vi "Set FP Origin.vi"(8 "error in":errorcluster, 11 "VI ref in":refnum<vi>) -> (0 "error out":errorcluster, 3 "VI Ref out":refnum<vi>)   [LabVIEW 2021, in "Utility.lvlib"]
uses:
  Utility.lvlib
  <vilib>/Utility/miscctls.llb/LVPointTypeDef.ctl
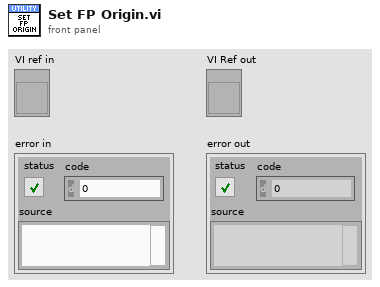
[diagram p1: front panel]
types:
  T1 = typedef "LVPointTypeDef.ctl" = cluster{"Horizontal":i16, "Vertical":i16}
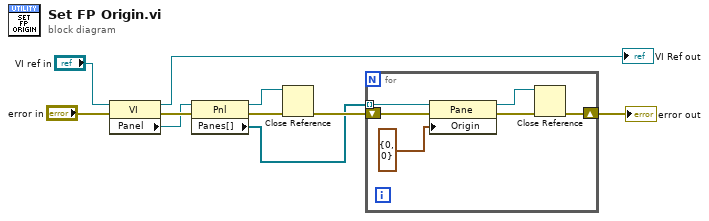
[diagram p0: block diagram]
diagram:
  n1 = property class="VI"(reference="VI ref in", error in="error in") -> (reference out=→"VI Ref out":refnum<vi>, error out=w6:errorcluster, "Panel"=w3:refnum<vi>)
  n2 = property class="Pnl"(reference=w3, error in=w6) -> (reference out=w4:refnum<vi>, error out=w8:errorcluster, "Panes[]"=w2:refnum<vi>[])
  n3 = Close Reference(reference=w4, error in (no error)=w8) -> (error out=w9:errorcluster)
  n4 = for {
    tunnel: w2 -> [w13] mode=indexing
    shift-right: [w14] -> w10
    shift-left: w9 -> [w16]
    n5 = property class="Pane"(reference=w13, error in=w16, "Origin"=T1 {"Horizontal"=0, "Vertical"=0}) -> (reference out=w11:refnum<vi>, error out=w15:errorcluster)
    n6 = Close Reference(reference=w11, error in (no error)=w15) -> (error out=w14:errorcluster)
  }
  "error out" <- w10
